vi "test xctrl.vi"() -> ()   [LabVIEW 2009]
uses:
  <vilib>/userDefined/High Color/IMAQdx.ctl
  XDisplay/POLARIS IMAQ Display.xctl
  IMAQdx Cam/IMAQdx Cam.lvclass
  XDisplay/Properties/ImageSource.ctl
  Analyze Classes/Analyze Fluence/Analyze Fluence.lvclass
panel:
  out "Max Fluence":dbl
  in  "Energy J":dbl
  out "error out":errorcluster
  in  "Prefix":string
  in  "WorkDir":path=path "D:/Test XDisplay images"
  out "POLARIS IMAQ Display":cluster{"Image":T1}(xcontrol)
  in  "stop":bool
  in  "Camera Name":T2="JustageCam"
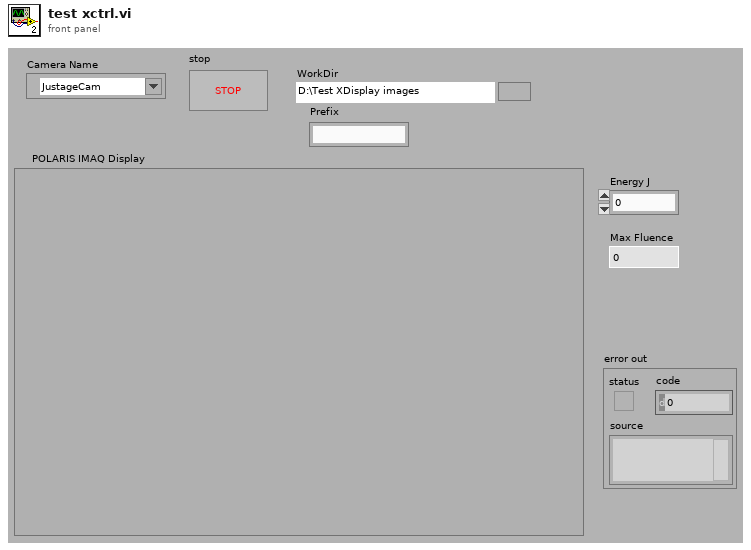
[diagram p1: front panel]
types:
  T1 = typedef "IMAQ Image.ctl" = refnum<image>
  T2 = typedef "IMAQdx.ctl" = refnum<k21>
  T3 = typedef "Image Type" = u32
  T4 = typedef "POLARIS IMAQ Display.xctl/ImageSource.ctl" = enum16{"Camera", "File"}
  T5 = cluster{"Global Rectangle":i32[], "Contours":cluster{"Contour Type":u32, "ROI Type":u32, "Points":i32[]}[]}
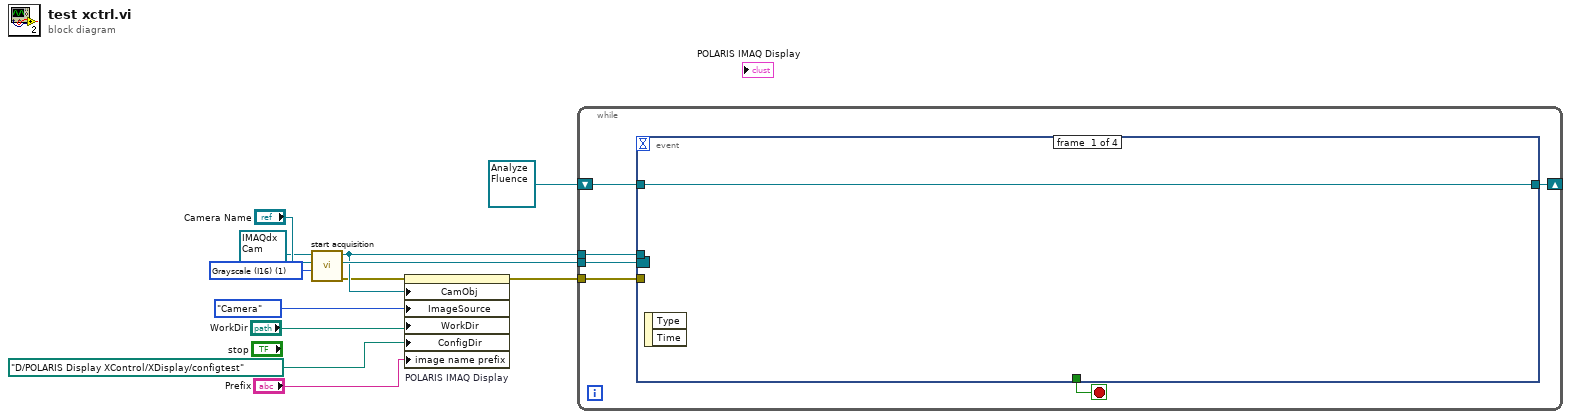
[diagram p0: block diagram]
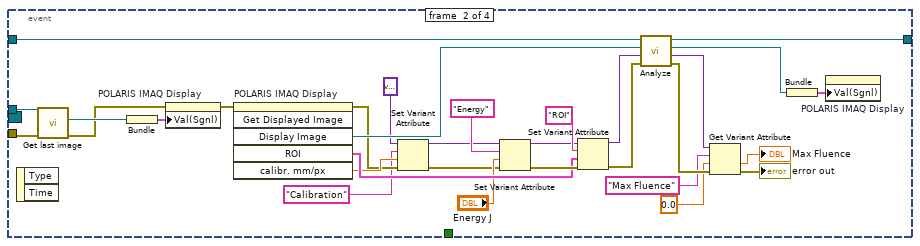
[diagram p2: hidden frame]
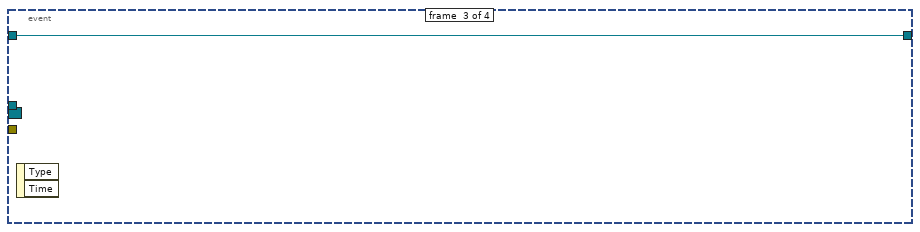
[diagram p3: hidden frame]
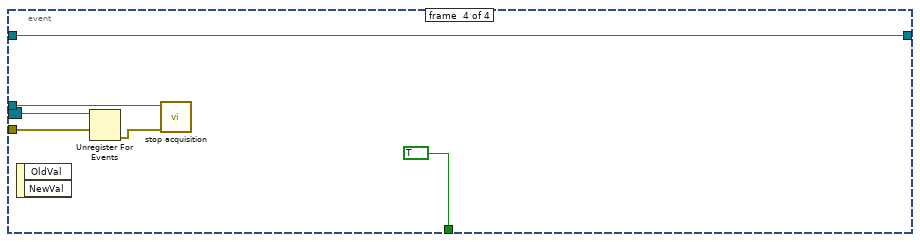
[diagram p4: hidden frame]
diagram:
  w4 = T3 1 items=["Grayscale (U8)", "Grayscale (I16)", "Grayscale (SGL)", "Complex (CSG)", "RGB (U32)", "HSL (U32)", "RGB (U64)", "Grayscale (U16)"] ("Image Type")
  n1 = call-dynamic "start acquisition.vi"("Image Type"=w4, "Camera Name"="Camera Name", "IMAQdx Cam in"=refnum<class "IMAQdx Cam.lvclass"> refnum ("IMAQdx Cam.lvclass")) -> ("error out"=w6:errorcluster, "Event Registration Refnum"=w11:refnum<event-registration>, "IMAQdx Cam out"=w7:refnum<class "IMAQdx Cam.lvclass">)  [unwired: 6 in]
  n2 = property on="POLARIS IMAQ Display" class="POLARIS IMAQ Display (strict)"(error in=w6, "CamObj"=w7, "ImageSource"=ImageSource."Camera", "WorkDir"="WorkDir", "ConfigDir"=path "D:/POLARIS Display XControl/XDisplay/configtest", "image name prefix"="Prefix") -> (error out=w5:errorcluster)  [unwired: 1 in, 1 out]
  n3 = while {
    tunnel: w7 -> [w17]
    tunnel: w11 -> [w16]
    tunnel: w5 -> [w15]
    shift-right: [w13] -> _
    shift-left: refnum<class "Analyze Fluence.lvclass"> refnum ("Analyze Fluence.lvclass") -> [w14]
    stop <- w18 stop-if-true
    n4 = event shown="[1] <Session Out>: FrameDone" {
      selector: w16 -> [_ _ _ w54]
      dyn-events: _ -> [_ _ _ _]
      timeout: _ -> [_ _ _ _]
      tunnel: [_ _ _ TRUE] -> w18
      tunnel: w17 -> [_ w50 _ w55]
      tunnel: w15 -> [_ w49 _ w53]
      tunnel: w14 -> [w19 w45 w51 w52]
      tunnel: [w19 w44 w51 w52] -> w13
      event #0 {
        n5 = event-data() -> ()  [unwired: 1 in, 2 out]
      }
      event #1 {
        n6 = event-data() -> ()  [unwired: 1 in, 2 out]
        n7 = call-dynamic "Get last image.vi"("error in (no error)"=w49, "IMAQdx Cam in"=w50) -> ("error out"=w46:errorcluster, "Image Out"=w48:T1)  [unwired: 7 in, 1 out]
        n8 = Bundle("Image Out"=w48) -> (w28:cluster{"Image Out":T1})  [unwired: 1 in]
        n9 = property on="POLARIS IMAQ Display" class="POLARIS IMAQ Display (strict)"(error in=w46, "Val(Sgnl)"=w28) -> (error out=w47:errorcluster)  [unwired: 1 in, 1 out]
        n10 = invoke on="POLARIS IMAQ Display" class="POLARIS IMAQ Display (strict)" method="Get Displayed Image"(error in=w47) -> (error out=w24:errorcluster, "Display Image"=w43:T1, "ROI"=w38:T5, "calibr. mm/px"=w25:sgl)  [unwired: 5 in, 2 out]
        n11 = Set Variant Attribute(Variant=variant ("variant"), name="Calibration", value=w25, error in=w24) -> (Variant out=w26:variant, error out=w23:errorcluster)  [unwired: 1 out]
        n12 = Set Variant Attribute(Variant=w26, name="Energy", value="Energy J", error in=w23) -> (Variant out=w39:variant, error out=w40:errorcluster)  [unwired: 1 out]
        n13 = Set Variant Attribute(Variant=w39, name="ROI", value=w38, error in=w40) -> (Variant out=w36:variant, error out=w37:errorcluster)  [unwired: 1 out]
        n14 = call-dynamic "Analyze.vi"("error in (no error)"=w37, "Parameters"=w36, "Image in"=w43, "Analyze Fluence in"=w45) -> ("error out"=w33:errorcluster, "Results"=w34:variant, "Image out"=w20:T1, "Analyze Fluence out"=w44:refnum<class "Analyze Fluence.lvclass">)  [unwired: 4 in]
        n15 = Get Variant Attribute(Variant=w34, name="Max Fluence", default value (empty Variant)=0.0 ("Energy J"), error in=w33) -> (value=→"Max Fluence":dbl, error out=→"error out":errorcluster)  [unwired: 2 out]
        n16 = Bundle("Image out"=w20) -> (w21:cluster{"Image out":T1})  [unwired: 1 in]
        n17 = property on="POLARIS IMAQ Display" class="POLARIS IMAQ Display (strict)"("Val(Sgnl)"=w21) -> ()  [unwired: 2 in, 2 out]
      }
      event #2 {
        n18 = event-data() -> ()  [unwired: 1 in, 2 out]
      }
      event #3 {
        n19 = event-data() -> ()  [unwired: 1 in, 2 out]
        n20 = Unregister For Events(event registration refnum=w54, error in=w53) -> (error out=w56:errorcluster)
        n21 = call-dynamic "stop acquisition.vi"("error in (no error)"=w56, "IMAQdx Cam in"=w55) -> ()  [unwired: 8 in, 2 out]
      }
    }
  }
